vi "serviceMode_disable.vi"(8 "error in (no error)":errorcluster, 11 "Thorlabs_OSA_64 in":refnum<class "OSA.lvclass">) -> (0 "error out":errorcluster, 3 "Thorlabs_OSA_64 out":refnum<class "OSA.lvclass">)   [LabVIEW 2010, in "OSA.lvclass"]
uses:
  OSA.lvclass
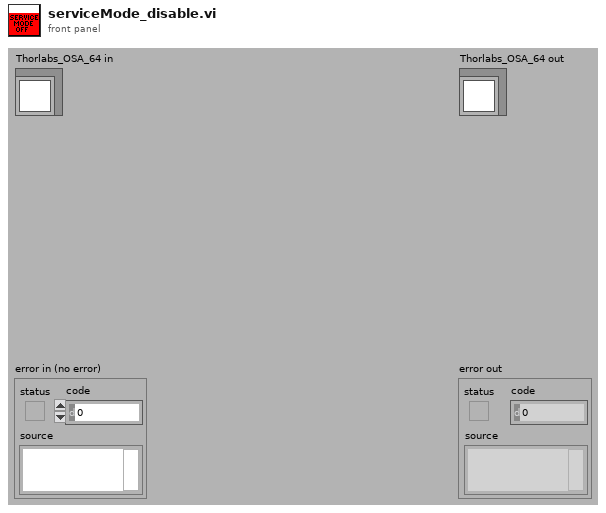
[diagram p1: front panel]
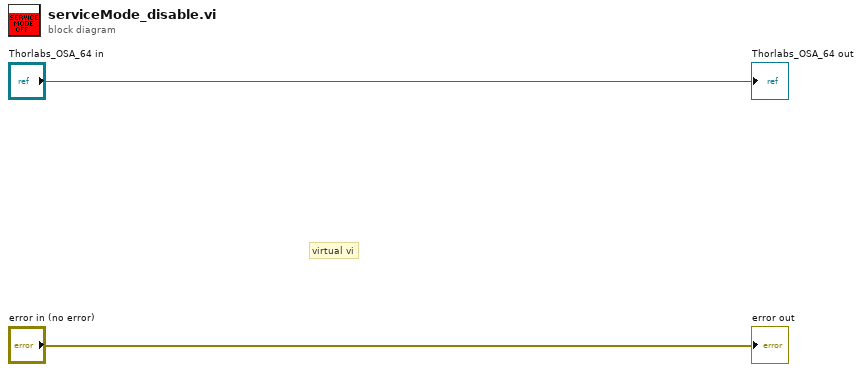
[diagram p0: block diagram]
diagram:
  # "virtual vi"
  "error out" <- "error in (no error)"
  "Thorlabs_OSA_64 out" <- "Thorlabs_OSA_64 in"
